vi "fix that xml.vi"(8 "error in (no error)":errorcluster, 10 "nw CD name":string, 11 "Path":path=path "C:/Program Files (x86)/National Instruments/LabVIEW 2015/ProjectTemplates/Source/NI VeriStand/Scripted Model Tool/Custom Device Scriptable Model Interface.xml") -> (0 "error out":errorcluster, 3 "Extra Pages":T1[](array[typedef]))   [LabVIEW 2014]
uses:
  TypDef/CD Wizard - Extra Page Name and GUID.ctl
  <vilib>/xml/Load XML File.vi
  <vilib>/xml/NI_XML.lvlib
  <resource>/objmgr/DOMUserDefRef.rc
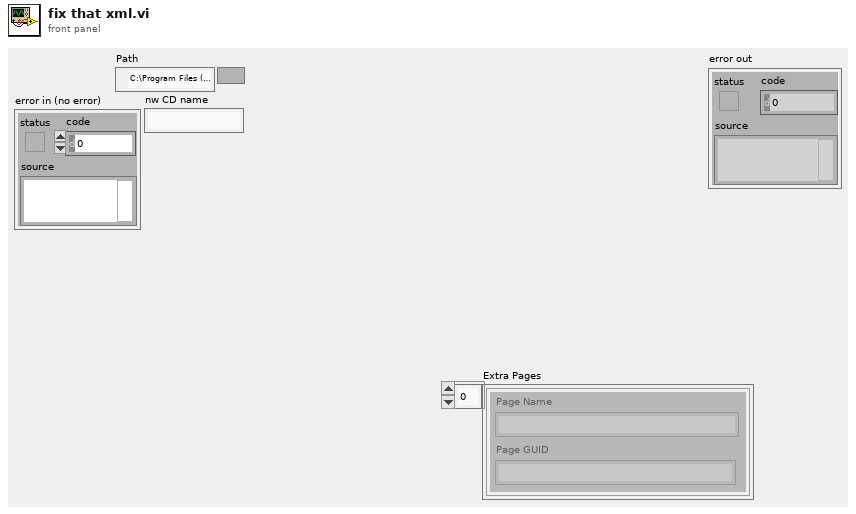
[diagram p1: front panel]
types:
  T1 = typedef "CD Wizard - Extra Page Name and GUID.ctl" = cluster{"Page Name":string, "Page GUID":string}
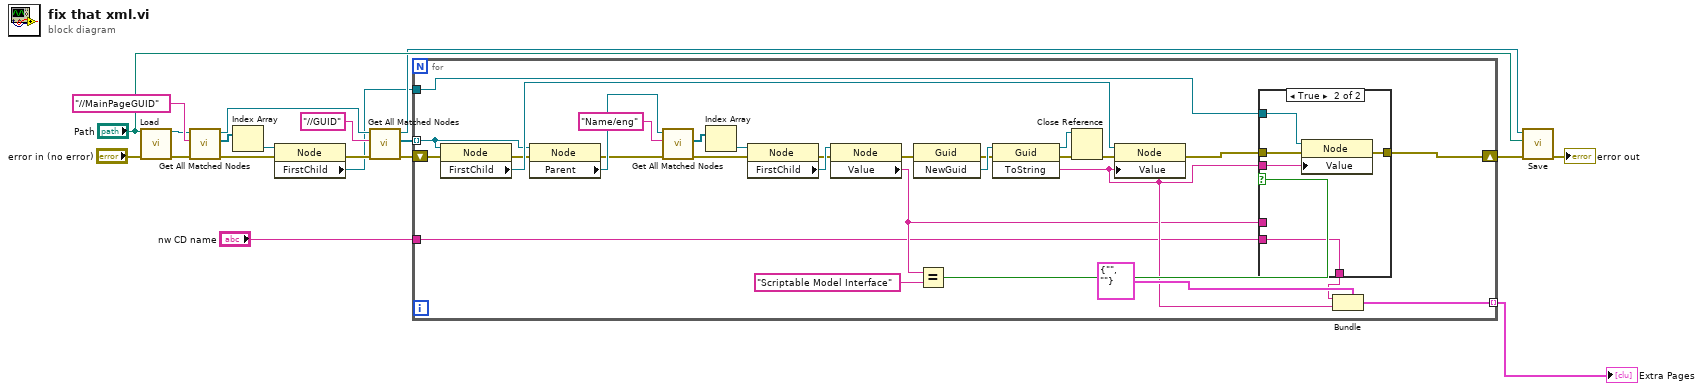
[diagram p0: block diagram]
diagram:
  n1 = call-poly <vilib>:"Load.vi"("path to XML document"="Path", "error in (no error)"="error in (no error)") -> ("DOM document out"=w13:refnum<k20>, "error out"=w14:errorcluster)  [unwired: 11 in, 1 out]
  n2 = call <vilib>:"Get All Matched Nodes.vi"("error in (no error)"=w14, "XPath expression"="//MainPageGUID", "node in"=w13) -> ("error out"=w15:errorcluster, "node result array"=w17:refnum<k20>[], "node out"=w12:refnum<k20>)  [unwired: 6 in]
  n3 = Index Array(array=w17) -> (element=w16:refnum<k20>)  [unwired: 1 in]
  n4 = property class="Node"(reference=w16, error in=w15) -> (error out=w4:errorcluster, "FirstChild"=w3:refnum<k20>)  [unwired: 1 out]
  n5 = call <vilib>:"Get All Matched Nodes.vi"("error in (no error)"=w4, "XPath expression"="//GUID", "node in"=w12) -> ("error out"=w10:errorcluster, "node result array"=w11:refnum<k20>[], "node out"=w8:refnum<k20>)  [unwired: 6 in]
  n6 = for {
    tunnel: w11 -> [w44] mode=indexing
    tunnel: [w47] -> w2 mode=indexing
    shift-right: [w27] -> w7
    shift-left: w10 -> [w35]
    tunnel: w3 -> [w25]
    tunnel: "nw CD name" -> [w20]
    n7 = property class="Node"(reference=w44, error in=w35) -> (error out=w39:errorcluster, "FirstChild"=w48:refnum<k20>)  [unwired: 1 out]
    n8 = property class="Node"(reference=w44, error in=w39) -> (error out=w40:errorcluster, "Parent"=w41:refnum<k20>)  [unwired: 1 out]
    n9 = call <vilib>:"Get All Matched Nodes.vi"("error in (no error)"=w40, "XPath expression"="Name/eng" ("Node Name"), "node in"=w41) -> ("error out"=w37:errorcluster, "node result array"=w42:refnum<k20>[])  [unwired: 6 in, 1 out]
    n10 = Index Array(array=w42) -> (element=w38:refnum<k20>)  [unwired: 1 in]
    n11 = property class="Node"(reference=w38, error in=w37) -> (error out=w34:errorcluster, "FirstChild"=w36:refnum<k20>)  [unwired: 1 out]
    n12 = property class="Node"(reference=w36, error in=w34) -> (error out=w33:errorcluster, "Value"=w22:string)  [unwired: 1 out]
    n13 = invoke class="Guid" method="NewGuid"(error in=w33) -> (error out=w32:errorcluster, "NewGuid"=w45:refnum<k24>)  [unwired: 2 in, 1 out]
    n14 = Equal?(x=w22, y="Scriptable Model Interface") -> (x = y?=w28:bool)
    n15 = invoke class="Guid" method="ToString"(reference=w45, error in=w32) -> (reference out=w46:refnum<k24>, error out=w31:errorcluster, "ToString"=w23:string)  [unwired: 1 in]
    n16 = Close Reference(reference=w46, error in (no error)=w31) -> (error out=w30:errorcluster)
    n17 = property class="Node"(reference=w48, error in=w30, "Value"=w23) -> (error out=w26:errorcluster)  [unwired: 1 out]
    n18 = case shown="True" w28 {
      tunnel: [w50 w54] -> w27
      tunnel: w26 -> [w50 w55]
      tunnel: w25 -> [_ w53]
      tunnel: w23 -> [_ w52]
      tunnel: w22 -> [w49 _]
      tunnel: [w49 w51] -> w21
      tunnel: w20 -> [_ w51]
      frame False {
      }
      frame True {
        n19 = property class="Node"(reference=w53, error in=w55, "Value"=w52) -> (error out=w54:errorcluster)  [unwired: 1 out]
      }
    }
    n20 = Bundle(cluster=T1 {"Page Name"="", "Page GUID"=""} ("Extra Page"), "Page Name"=w21, "Page GUID"=w23) -> (w47:T1)
  }
  "Extra Pages" <- w2
  n21 = call <vilib>:"Save.vi"("error in (no error)"=w7, "XML file path"="Path", "DOM document in"=w8) -> ("error out"=→"error out":errorcluster)  [unwired: 6 in, 2 out]
